vi "Shoot.vi"(5 "FirstCall?":bool, 7 "KickTarget":dbl[](array[numeric]), 8 "error in (no error)":errorcluster, 9 "Game":refnum<class "Game.lvclass">, 10 "Robot":refnum<class "Robot.lvclass">, 11 "KickToSkill in":refnum<class "KickToSkill.lvclass">) -> (0 "error out":errorcluster, 2 "Robot out":refnum<class "Robot.lvclass">, 3 "KickToSkill out":refnum<class "KickToSkill.lvclass">)   [LabVIEW 2023, in "KickToSkill.lvclass"]
uses:
  KickToSkill.lvclass
  Game_class/Game.lvclass
  Robot_class/Robot.lvclass
  Game_class/Game.lvclass/Game.ctl
  Parameters_class/Parameters.lvclass/Parameters.ctl
  Game_class/Read Parameters.lvclass.vi
  Parameters_class/Read KickForce.vi
  Parameters_class/Parameters.lvclass
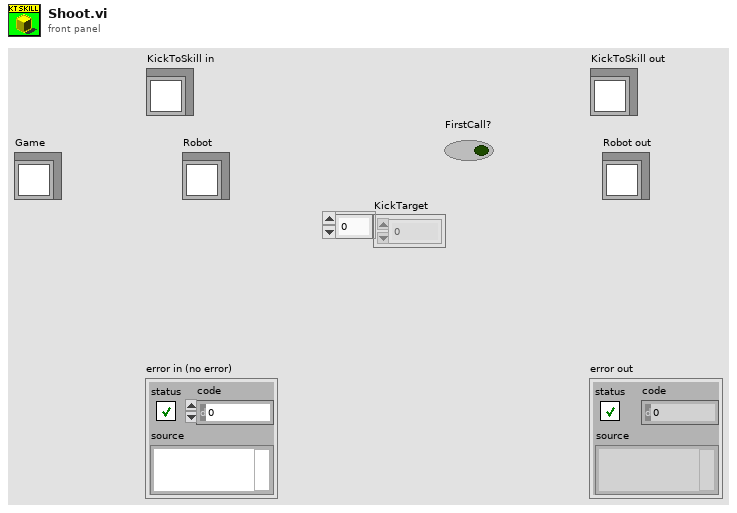
[diagram p1: front panel]
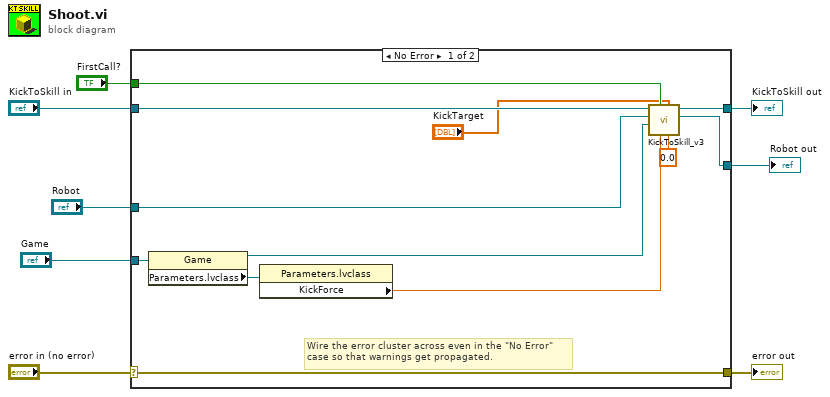
[diagram p0: block diagram]
diagram:
  n1 = case shown="No Error" "error in (no error)" {
    selector: "error in (no error)" -> [w20 w23]
    tunnel: [w20 w23] -> w7
    tunnel: [w19 w22] -> w5
    tunnel: "KickToSkill in" -> [w17 w22]
    tunnel: "FirstCall?" -> [w18 _]
    tunnel: "Game" -> [w16 _]
    tunnel: "Robot" -> [w14 w21]
    tunnel: [w12 w21] -> w1
    frame No Error {
      # "Wire the error cluster across even in the \"No Error\"\ncase so that warnings get propagated."
      n2 = property class="Game"(reference=w16) -> (reference out=w13:refnum<class "Game.lvclass">, "Parameters.lvclass"=w15:refnum<class "Parameters.lvclass">)  [unwired: 1 in, 1 out]
      n3 = property class="Parameters.lvclass"(reference=w15) -> ("KickForce"=w10:dbl)  [unwired: 1 in, 2 out]
      n4 = call "KickToSkill_v3.vi"("kick_z"=0.0, "KickTarget"="KickTarget", "kick_x"=w10, "firstCall?"=w18, "Game"=w13, "Robot"=w14, "KickToSkill in"=w17) -> ("Robot out"=w12:refnum<class "Robot.lvclass">, "KickToSkill out"=w19:refnum<class "KickToSkill.lvclass">)  [unwired: 2 in, 1 out]
    }
    frame Error {
    }
  }
  "error out" <- w7
  "KickToSkill out" <- w5
  "Robot out" <- w1
